vi "DAQ.AIData.FGV.vi"(7 "Action":T1, 8 "Error In":errorcluster, 11 "Data In":dbl[][](array[numeric])) -> (0 "Error Out":errorcluster, 3 "Data Out":dbl[][](array[numeric]))   [LabVIEW 2017, in "DAQ.lvlib"]
uses:
  DAQ.lvlib
  DAQ.AIData.FGV.Action.ctl
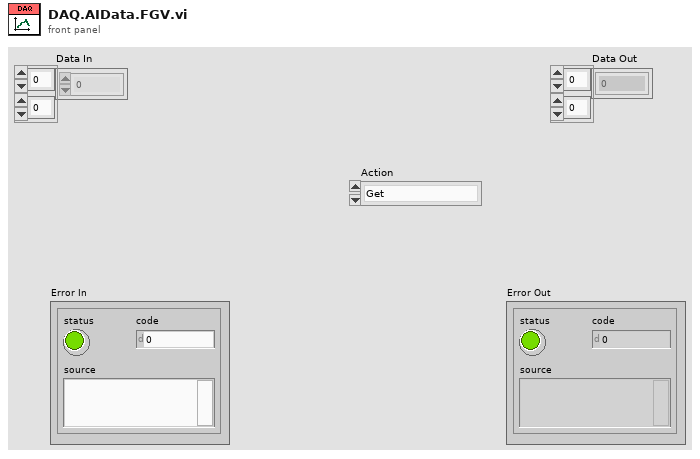
[diagram p1: front panel]
types:
  T1 = typedef "DAQ.lvlib/DAQ.AIData.FGV.Action.ctl" = enum16{"Get", "Add", "Clear"}
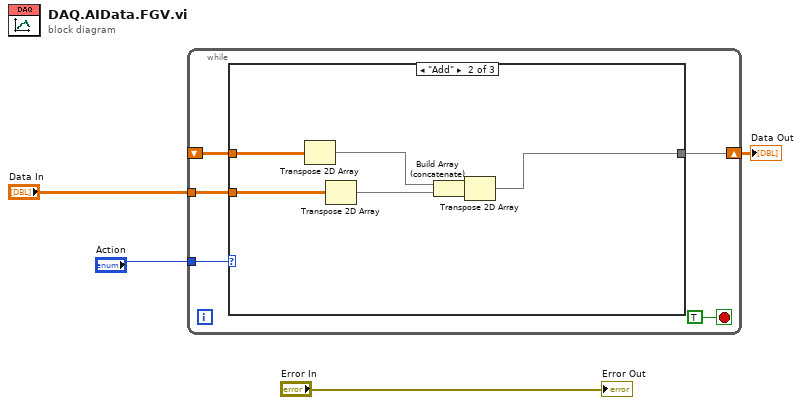
[diagram p0: block diagram]
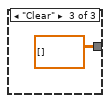
[diagram p3: hidden frame]
diagram:
  n1 = while {
    tunnel: "Action" -> [w8]
    shift-right: [w5] -> w2
    shift-left: _ -> [w7]
    tunnel: "Data In" -> [w6]
    stop <- TRUE stop-if-true
    n2 = case shown="\"Add\"" w8 {
      tunnel: w7 -> [w10 w13 _]
      tunnel: w6 -> [_ w12 _]
      tunnel: [w10 w11 dbl[][] []] -> w5
      frame "Get" {
      }
      frame "Add" {
        n3 = Transpose 2D Array(2D array=w13) -> (transposed array=w15:dbl[][])
        n4 = Transpose 2D Array(2D array=w12) -> (transposed array=w14:dbl[][])
        n5 = Build Array (concatenate)(w15, w14) -> (w16:dbl[][])
        n6 = Transpose 2D Array(2D array=w16) -> (transposed array=w11:dbl[][])
      }
      frame "Clear" {
      }
    }
  }
  "Data Out" <- w2
  "Error Out" <- "Error In"
